vi "3lampice.vi"(5 "Cluster":T1) -> (1 "Lampice":T2)   [LabVIEW 2019]
doc: "Brojevna kontrola koliko od 3 lampice u klasteru da svetli"
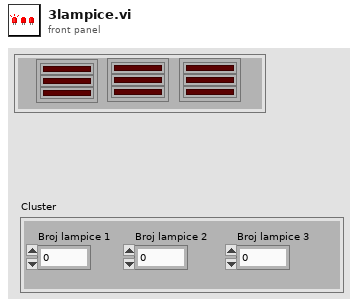
[diagram p1: front panel]
types:
  T1 = cluster{"Broj lampice 1":dbl, "Broj lampice 2":dbl, "Broj lampice 3":dbl}
  T2 = cluster{"3 lampice":cluster{"led3coffee1":bool, "led2coffee1":bool, "led1coffee1":bool}, "3 lampice 2":cluster{"led3coffee1":bool, "led2coffee1":bool, "led1coffee1":bool}, "3 lampice 3":cluster{"led3coffee1":bool, "led2coffee1":bool, "led1coffee1":bool}}
  T3 = cluster{cluster{bool, bool, bool}, cluster{bool, bool, bool}, cluster{bool, bool, bool}}
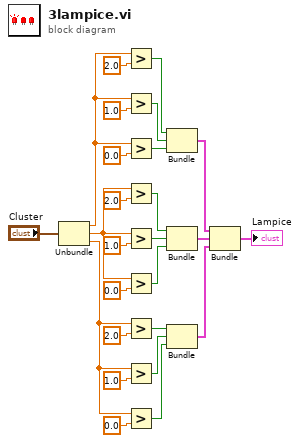
[diagram p0: block diagram]
diagram:
  n1 = Unbundle("Cluster") -> ("Broj lampice 1"=w3:dbl, "Broj lampice 2"=w2:dbl, "Broj lampice 3"=w1:dbl)
  n2 = Greater?(x=w3, y=2.0) -> (0:w13:bool)
  n3 = Greater?(x=w3, y=1.0) -> (0:w11:bool)
  n4 = Greater?(x=w3, y=0.0) -> (0:w9:bool)
  n5 = Greater?(x=w2, y=2.0) -> (0:w25:bool)
  n6 = Greater?(x=w2, y=1.0) -> (0:w23:bool)
  n7 = Greater?(x=w2, y=0.0) -> (0:w21:bool)
  n8 = Greater?(x=w1, y=2.0) -> (0:w19:bool)
  n9 = Greater?(x=w1, y=1.0) -> (0:w17:bool)
  n10 = Greater?(x=w1, y=0.0) -> (0:w15:bool)
  n11 = Bundle(w13, w11, w9) -> (w8:cluster{bool, bool, bool})  [unwired: 1 in]
  n12 = Bundle(w25, w23, w21) -> (w7:cluster{bool, bool, bool})  [unwired: 1 in]
  n13 = Bundle(w19, w17, w15) -> (w6:cluster{bool, bool, bool})  [unwired: 1 in]
  n14 = Bundle(w8, w7, w6) -> (→"Lampice":T3)  [unwired: 1 in]
